vi "fpga_Integration Core.vi"(7 "integrate?":bool=TRUE, 8 "input valid":bool=TRUE, 9 "dt/T":fxp<+/-,32,1>, 11 "previous integrated value":fxp<+,32,0>) -> (0 "output valid":bool, 3 "integrated value out":fxp<+,32,0>)   [LabVIEW 2012, in "NI_EP_Protection_FPGA.lvlib"]
uses:
  <vilib>/addons/Electrical Power/Protection/NI_EP_Protection_FPGA.lvlib
  <vilib>/rvi/FXPMathLib/FxpAdd/XNode/nifxpmath_Add.xnode
  <vilib>/rvi/FXPMathLib/sim/FxpSim.dll
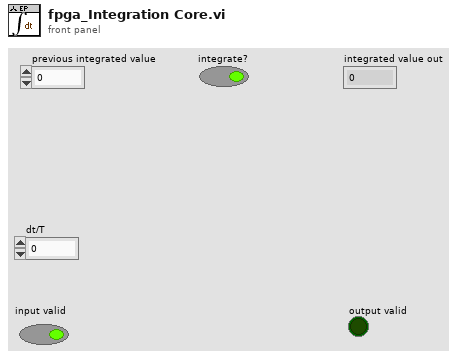
[diagram p1: front panel]
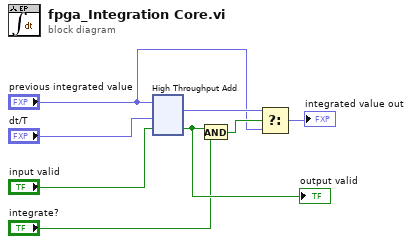
[diagram p0: block diagram]
diagram:
  n1 = xnode ("High Throughput Add")("x"="previous integrated value", "y"="dt/T", "input valid"="input valid") -> ("x+y"=w8:fxp<+,32,0>, "output valid"=w7:bool)  [unwired: 1 in, 1 out]
  "output valid" <- w7
  n2 = And(x=w7, y="integrate?") -> (x .and. y?=w3:bool)
  n3 = Select(t=w8, s=w3, f="previous integrated value") -> (s? t:f=→"integrated value out":fxp<+,32,0>)
